vi "Close.vi"(8 "error in (no error)":errorcluster, 9 "timeout ms (5000)":i32=5000, 11 "WebSocket Connection in":refnum<k5>) -> (0 "error out":errorcluster, 3 "WebSocket Connection in":refnum<k5>)   [LabVIEW 2013, in "WebSockets.lvlib"]
doc: "Sends the shutdown opcode to the TCP socket. This VI will run even if an upstream error has occurred.\n\nNote: This does not close the TCP connection as you may want to wait for the shutdown opcode to be received from the client."
uses:
  WebSockets.lvlib
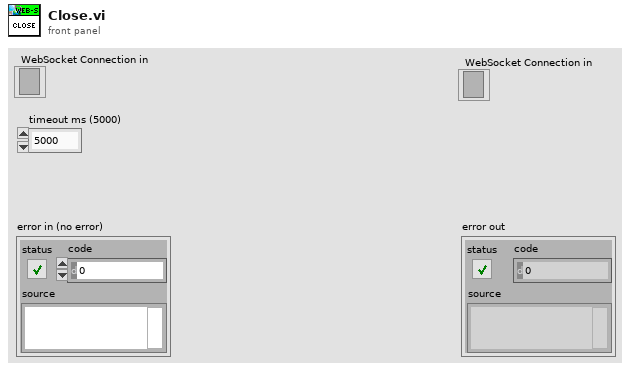
[diagram p1: front panel]
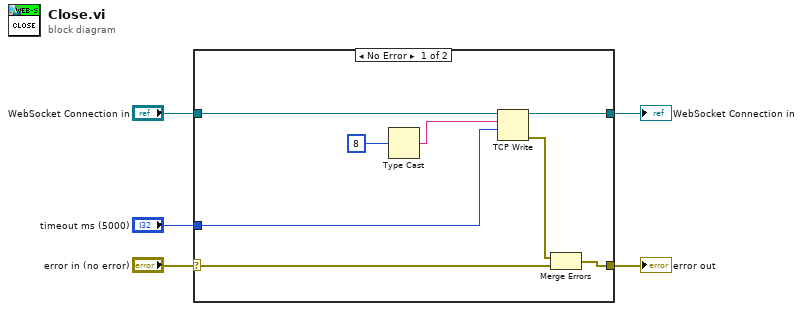
[diagram p0: block diagram]
diagram:
  n1 = case shown="No Error" "error in (no error)" {
    selector: "error in (no error)" -> [w9 w15]
    tunnel: [w10 w15] -> w4
    tunnel: [w13 w14] -> w2
    tunnel: "WebSocket Connection in" -> [w12 w14]
    tunnel: "timeout ms (5000)" -> [w11 _]
    frame No Error {
      n2 = Type Cast(x=u8 8) -> (*(type *) &x=w6:string)  [unwired: 1 in]
      n3 = TCP Write(connection ID=w12, data in=w6, 9:w11) -> (connection ID out=w13:refnum<k5>, error out=w8:errorcluster)  [unwired: 1 in, 1 out]
      n4 = Merge Errors(w8, w9) -> (w10:errorcluster)
    }
    frame Error {
    }
  }
  "WebSocket Connection in" <- w2
  "error out" <- w4
